vi "offset t graph.vi"(10 "t0":dbl=-1.0 format="%#_13g", 11 "graphs":cluster{dbl[], "Best Linear Fit":dbl[]}[](array[cluster])) -> (2 "t0 out":dbl, 3 "t offset graphs":cluster{dbl[], "Best Linear Fit":dbl[]}[](array[cluster]))   [LabVIEW 2017]
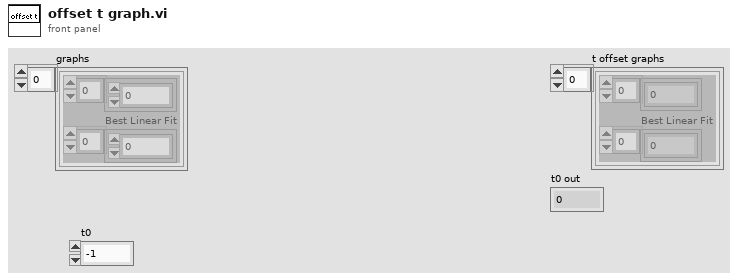
[diagram p1: front panel]
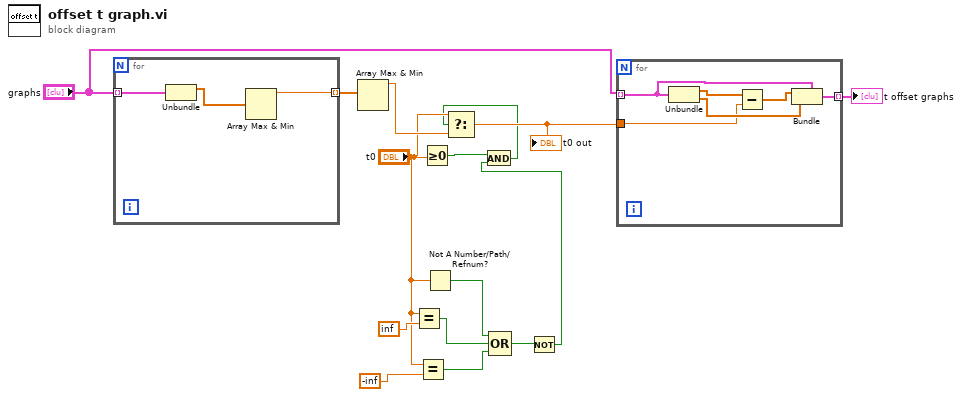
[diagram p0: block diagram]
diagram:
  n1 = for {
    tunnel: "graphs" -> [w18] mode=indexing
    tunnel: [w16] -> w15 mode=indexing
    n2 = Unbundle(w18) -> (w17:dbl[])  [unwired: 1 out]
    n3 = Array Max & Min(array=w17) -> (max value=w16:dbl)  [unwired: 3 out]
  }
  n4 = Array Max & Min(array=w15) -> (max value=w14:dbl)  [unwired: 3 out]
  n5 = Equal?(x="t0", y=inf) -> (x = y?=w5:bool)
  n6 = Equal?(x="t0", y=-inf) -> (x = y?=w4:bool)
  n7 = Greater Or Equal To 0?(x="t0") -> (x >= 0?=w10:bool)
  n8 = Not A Number/Path/Refnum?(number/path/refnum="t0") -> (NaN/Path/Refnum?=w6:bool)
  n9 = Compound Arithmetic op=OR(w6, w5, w4) -> (w3:bool)
  n10 = Not(x=w3) -> (.not. x?=w2:bool)
  n11 = And(x=w10, y=w2) -> (x .and. y?=w1:bool)
  n12 = Select(t="t0", s=w1, f=w14) -> (s? t:f=w12:dbl)
  "t0 out" <- w12
  n13 = for {
    tunnel: "graphs" -> [w23] mode=indexing
    tunnel: w12 -> [w20]
    tunnel: [w19] -> w11 mode=indexing
    n14 = Unbundle(w23) -> (w24:dbl[], "Best Linear Fit"=w21:dbl[])
    n15 = Subtract(x=w24, y=w20) -> (x-y=w22:dbl[])
    n16 = Bundle(cluster=w23, w22, "Best Linear Fit"=w21) -> (w19:cluster{dbl[], "Best Linear Fit":dbl[]})
  }
  "t offset graphs" <- w11
